vi "Script_Timing_Extract_Table_From_Text_HardCoded.vi"(8 "error in (no error)":errorcluster) -> (0 "error out":errorcluster)   [LabVIEW 2018]
uses:
  controls/TIMING_Mandatory_Items.ctl
panel:
  out "Mandatory Items Output":T1={"Script Name"="", "HSDIO Delay"=60.0, "Shutter Duration before"=50.0, "Shutter Duration after"=50.0, "Filter Tau"=2.0, "Trapping Delay"=600.0, "Trapping Duration"=300.0, "Emtyping Duration"=1000.0} {"Shutter Duration after" min=2.0 max=100000.0; "HSDIO Delay" min=60.0 max=100.0; "Shutter Duration before" min=2.0 max=100000.0; "Filter Tau" min=1000.0 max=2000.0; "Trapping Delay" min=2.0; "Emtyping Duration" min=2.0 format="%#_8g"; "Trapping Duration" min=2.0}
  in  "Mandatory Items":T1={"Script Name"="", "HSDIO Delay"=60.0, "Shutter Duration before"=50.0, "Shutter Duration after"=50.0, "Filter Tau"=2.0, "Trapping Delay"=600.0, "Trapping Duration"=300.0, "Emtyping Duration"=1000.0} {"Shutter Duration after" min=2.0 max=100000.0; "HSDIO Delay" min=60.0 max=100.0; "Shutter Duration before" min=2.0 max=100000.0; "Filter Tau" min=1000.0 max=2000.0; "Trapping Delay" min=2.0; "Emtyping Duration" min=2.0 format="%#_8g"; "Trapping Duration" min=2.0}
  in  "Table of Waits":string[](array[string])=["949940", "48000", "2000", "600", "300", "2000", "47100", "3950000", "1200", "1200", "1000000", "1000", "1000000", "2000"]
  in  "Table of Wfms":string[](array[string])=["AutLaserOn", "AutLaserOnFilterOff", "AutLaserOnFilterOffTrapStart", "AutLaserOnFilterOffTrapStop", "AutLaserOnFilterOn", "AutLaserOff", "Excit", "Excit", "Acq", "FilterOff", "FilterOffEmptyingStart", "FilterOffEmptyingStop", "Zeros"]
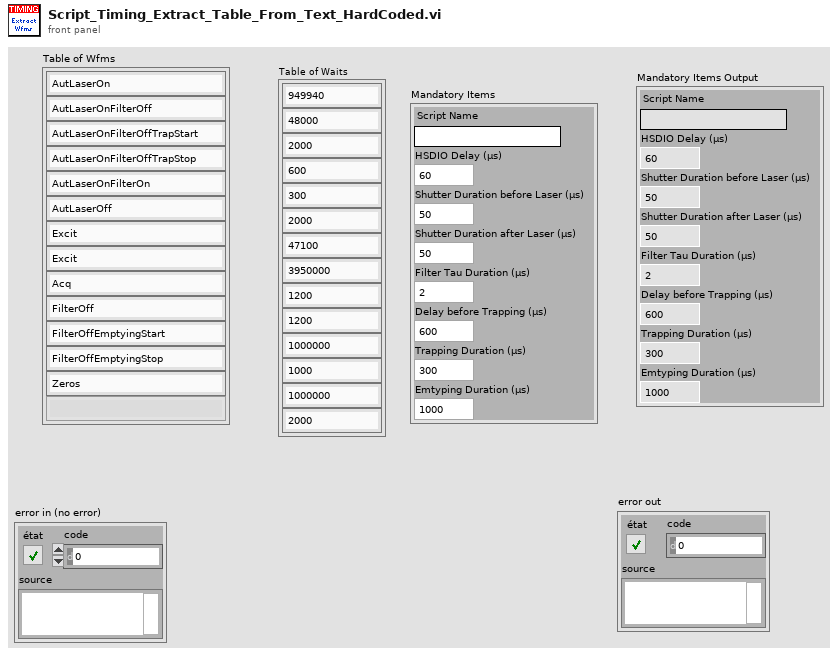
[diagram p1: front panel]
types:
  T1 = typedef "TIMING_Mandatory_Items.ctl" = cluster{"Script Name":string, "HSDIO Delay":dbl, "Shutter Duration before":dbl, "Shutter Duration after":dbl, "Filter Tau":dbl, "Trapping Delay":dbl, "Trapping Duration":dbl, "Emtyping Duration":dbl}
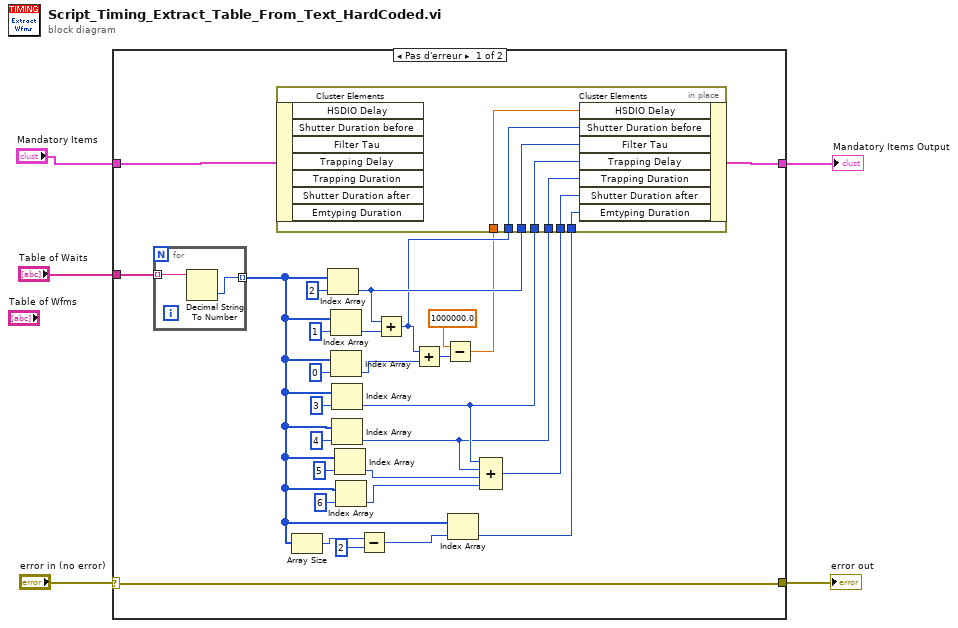
[diagram p0: block diagram]
diagram:
  n1 = case shown="Pas d'erreur" "error in (no error)" {
    selector: "error in (no error)" -> [w33 w44]
    tunnel: [w33 w44] -> w5
    tunnel: "Mandatory Items" -> [w32 w43]
    tunnel: "Table of Waits" -> [w25 _]
    tunnel: [w16 w43] -> w1
    frame No Error {
      n2 = for {
        tunnel: [w34] -> w9 mode=indexing
        tunnel: w25 -> [w35] mode=indexing
        n3 = Decimal String To Number(string=w35) -> (number=w34:i32)  [unwired: 2 in, 1 out]
      }
      n4 = Array Size(array=w9) -> (size(s)=w7:i32)
      n5 = Index Array(array=w9, index=2 ("indice")) -> (element=w29:i32)
      n6 = Index Array(array=w9, index=1 ("indice")) -> (element=w28:i32)
      n7 = Index Array(array=w9, index=0 ("indice")) -> (element=w15:i32)
      n8 = Index Array(array=w9, index=3 ("indice")) -> (element=w21:i32)
      n9 = Index Array(array=w9, index=4 ("indice")) -> (element=w20:i32)
      n10 = Index Array(array=w9, index=5 ("indice")) -> (element=w19:i32)
      n11 = Index Array(array=w9, index=6 ("indice")) -> (element=w18:i32)
      n12 = Subtract(x=w7, y=2) -> (x-y=w10:i32)
      n13 = Add(x=w29, y=w28) -> (x+y=w14:i32)
      n14 = Add(x=w14, y=w15) -> (x+y=w13:i32)
      n15 = Subtract(x=1000000.0, y=w13) -> (x-y=w12:dbl)
      n16 = Index Array(array=w9, index=w10) -> (element=w8:i32)
      n17 = Compound Arithmetic op=ADD(w21, w20, w19, w18) -> (w17:i32)
      n18 = in-place {
        in-place-border: w29 -> [w42]
        in-place-border: w14 -> [w41]
        in-place-border: w21 -> [w40]
        in-place-border: w20 -> [w39]
        in-place-border: w17 -> [w38]
        in-place-border: w12 -> [w37]
        in-place-border: w8 -> [w36]
        n19 = in-place-cluster #1(w32) -> ()  [unwired: 7 out]
        n20 = in-place-cluster #1("HSDIO Delay"=w37, "Shutter Duration before"=w41, "Filter Tau"=w42, "Trapping Delay"=w40, "Trapping Duration"=w39, "Shutter Duration after"=w38, "Emtyping Duration"=w36) -> (w16:T1)
      }
    }
    frame Error {
    }
  }
  "error out" <- w5
  "Mandatory Items Output" <- w1
